vi "W vs Z main4h.vi"() -> ()   [LabVIEW 2016]
panel:
  out "cursor X's":dbl[](array[numeric])
  out "Contains waist?":bool[](array[boolean])
  out "FWHM":dbl[](array[numeric])
  out "min w":dbl[](array[numeric])
  out "min z":dbl[](array[numeric])
  out "w Matrix":dbl[][](array[numeric])
  out "Z Matrix":dbl[][](array[numeric])
  out "Number of lenses":i32
  in  "Lens Focal lengths":dbl[](array[numeric]) format="%.3f"
  in  "FWHM(T)?":bool
  out "Cursor List":T1(array[cluster]) {"Location"."Y" format="%.2f"; "Location"."X" format="%.2f"}
  in  "z stop":dbl=1000.0 format="%.2f"
  in  "N steps":i32=500
  out "Q start":cdb format="%.4f"
  out "W vs Z":cluster{dbl[], dbl[]}[](graph)=[{array[5001 elements], array[5001 elements]}, {array[5000 elements], array[5000 elements]}, {array[5000 elements], array[5000 elements]}, {array[5001 elements], array[5001 elements]}, {array[5001 elements], array[5001 elements]}, {array[5001 elements], array[5001 elements]}, {[6000.0], [0.9936206464518128]}]
  in  "beam radius(w)":dbl=0.6 format="%.5f"
  in  "Radius of Curvature":dbl=inf format="%.2f"
  in  "Wavelength":dbl=0.00035 format="%.6f"
  in  "z start":dbl format="%.2f"
  # "All values are entered in mm"
  # "w is the 1/e field radius"
  # "w x 1.18 to get FWHM of the Intensity"
  # "For more lenses\njust create more \ncursors here"
  # "Zs plotted above. Each row is a segment between adjacent lenses"
  # "Ws plotted above. Each row is a segment between adjacent lenses"
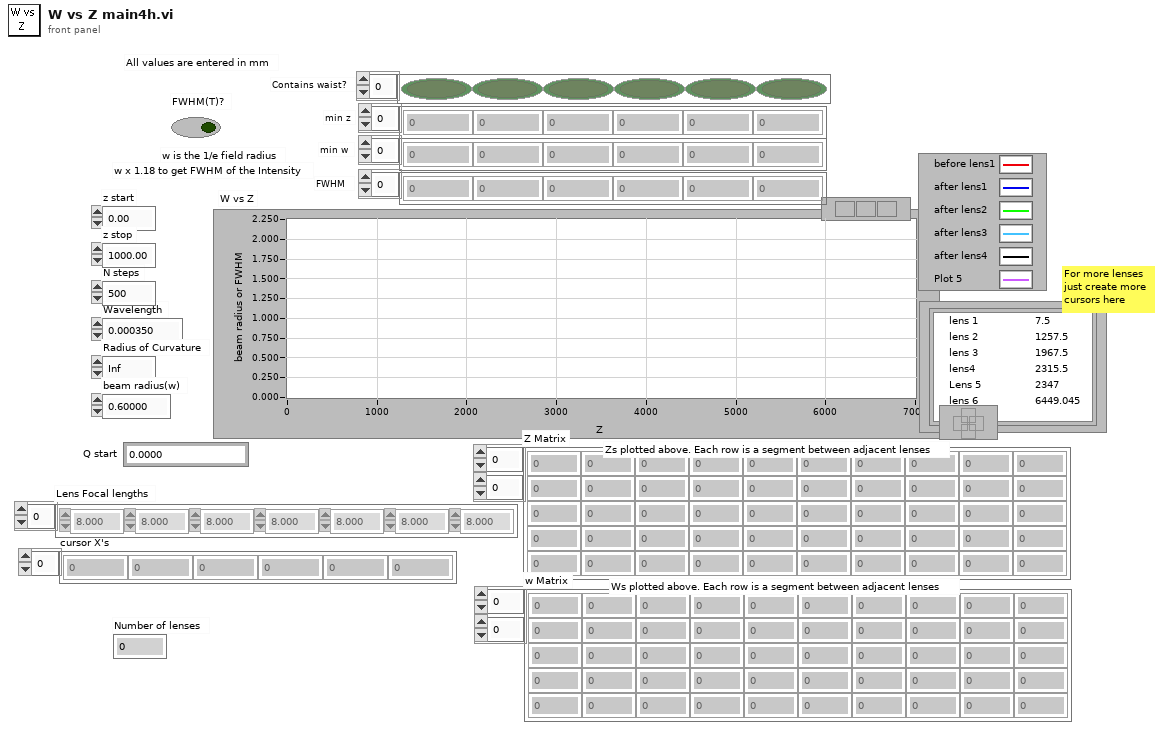
[diagram p1: front panel]
types:
  T1 = cluster{"Name":string, "Color":u32, "Hair Style":u8, "Point Style":u8, "Name Visible":bool, "Trackable":bool, "Lock Style":u32, "Plot Number":u32, "Marker Index":i32, "Location":cluster{"X":dbl, "Y":dbl}}[]
  T2 = cluster{"Name":string, "Color":u32, "Style":u8, "Point Style":u8, "Name Visible":bool, "Allow Drag":bool, "Lock Style":u32, "Plot":u32, "Index":i32, "Position":cluster{"X":dbl, "Y":dbl}}[]
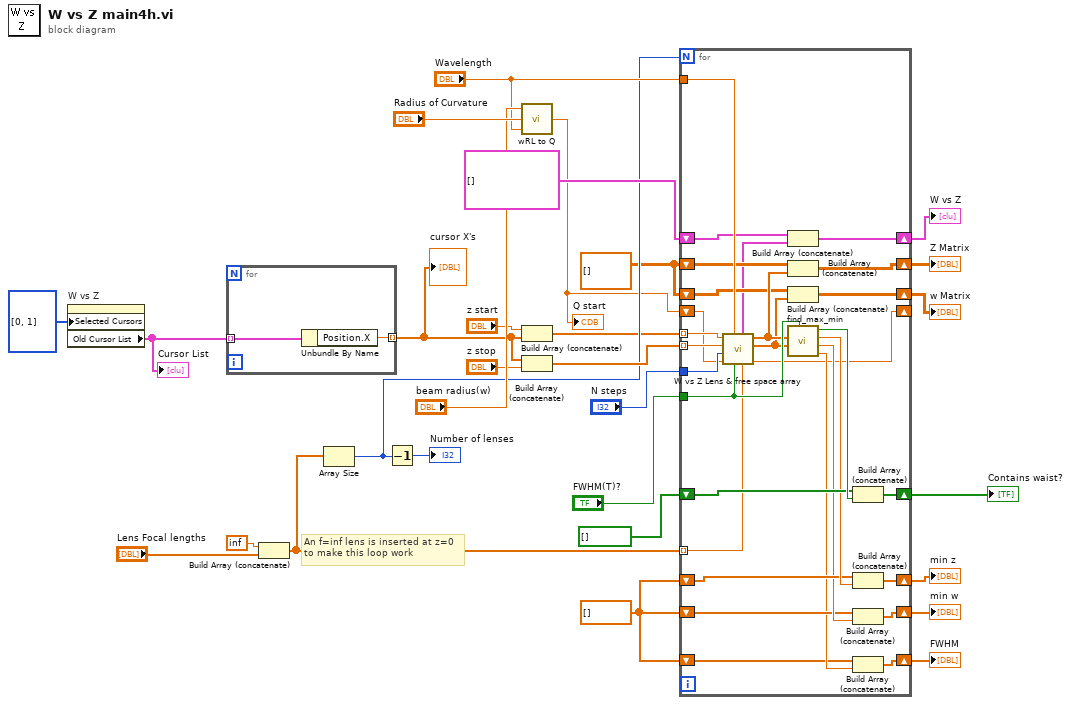
[diagram p0: block diagram]
diagram:
  w9 = dbl[] []
  w8 = dbl[][] []
  # "An f=inf lens is inserted at z=0\nto make this loop work"
  n1 = property on="W vs Z" class="XYGraph (strict)"("Selected Cursors"=u32[] [0, 1]) -> ("Old Cursor List"=w2:T2)  [unwired: 2 in, 2 out]
  "Cursor List" <- w2
  n2 = for {
    tunnel: w2 -> [w31] mode=indexing
    tunnel: [w30] -> w1 mode=indexing
    n3 = Unbundle By Name(w31) -> ("Position.X"=w30:dbl)
  }
  "cursor X's" <- w1
  n4 = Build Array (concatenate)(inf, "Lens Focal lengths") -> (w11:dbl[])
  n5 = Array Size(array=w11) -> (size(s)=w14:i32)
  n6 = Decrement(x=w14) -> (x-1=→"Number of lenses":i32)
  n7 = call "wRL to Q.vi"("Wavelength"="Wavelength", "Radius of Curvature"="Radius of Curvature", "beam radius(w)"="beam radius(w)") -> ("Q"=w10:cdb)
  "Q start" <- w10
  n8 = Build Array (concatenate)("z start", w1) -> (w3:dbl[])
  n9 = Build Array (concatenate)(w1, "z stop") -> (w21:dbl[])
  n10 = for {
    N: w14 -> [_]
    tunnel: "N steps" -> [w60]
    tunnel: w21 -> [w59] mode=indexing
    tunnel: w3 -> [w58] mode=indexing
    tunnel: "Wavelength" -> [w57]
    tunnel: "FWHM(T)?" -> [w56]
    shift-right: [w55] -> w5
    shift-left: bool[] [] -> [w53]
    shift-right: [w51] -> w18
    shift-left: w9 -> [w50]
    shift-right: [w48] -> w17
    shift-left: w9 -> [w47]
    shift-right: [w35] -> w16
    shift-left: w9 -> [w45]
    shift-right: [w43] -> w22
    shift-left: w8 -> [w42]
    shift-right: [w40] -> w19
    shift-left: w8 -> [w39]
    shift-right: [w38] -> _
    shift-left: w10 -> [w37]
    tunnel: w11 -> [w36] mode=indexing
    shift-right: [w33] -> w23
    shift-left: cluster{dbl[], dbl[]}[] [] -> [w32]
    n11 = call "W vs Z Lens & free space array.vi"("lens focal length"=w36, "FWHM(T)?"=w56, "Wavelength"=w57, "Q in"=w37, "N steps"=w60, "z stop"=w59, "z start"=w58) -> ("Q out"=w38:cdb, "w/FWHM Array"=w41:dbl[], "Z Array"=w44:dbl[], "W/FWHM vs Z"=w34:cluster{dbl[], dbl[]})  [unwired: 1 out]
    n12 = Build Array (concatenate)(w32, w34) -> (w33:cluster{dbl[], dbl[]}[])
    n13 = Build Array (concatenate)(w42, w44) -> (w43:dbl[][])
    n14 = Build Array (concatenate)(w39, w41) -> (w40:dbl[][])
    n15 = call "find_max_min.vi"("FWHM(T)?"=w56, "w Array"=w41, "z Array"=w44) -> ("FWHM"=w46:dbl, "min w"=w49:dbl, "min  z"=w52:dbl, "contains waist?"=w54:bool)  [unwired: 5 in]
    n16 = Build Array (concatenate)(w53, w54) -> (w55:bool[])
    n17 = Build Array (concatenate)(w50, w52) -> (w51:dbl[])
    n18 = Build Array (concatenate)(w47, w49) -> (w48:dbl[])
    n19 = Build Array (concatenate)(w45, w46) -> (w35:dbl[])
  }
  "W vs Z" <- w23
  "Z Matrix" <- w22
  "w Matrix" <- w19
  "min z" <- w18
  "min w" <- w17
  "FWHM" <- w16
  "Contains waist?" <- w5
